vi "string parse mathematica assosiated array.vi"(7 "action":T2=enum."parse string", 10 "map IN":map{T1, dbl}(c390), 11 "String in":string="8061 -> <|\n\"\\[Zeta]\" -> 0.029251354442, \n\"\\[Tau]1\" -> 0.014634751206, \n\"\\[Tau]S\" -> 0.003873958746, \n\"\\[Tau]N\" -> 0.000007000487,\n\"\\[Tau]C\" -> 0.006827504775,\n\"\\[Kappa]0\" -> 0.000000056438,\n\"mm1\" -> 0.000000000000,\n\"mm2\" -> 0.000000000000,\n\"mm3\" -> 0.000000000000,\n\"T\" ->  5.820000000000,\n\"B\" -> 12.000000000000,\n\"\\[Theta]\" -> 0.000000000000\n|>, \n\n ") -> (2 "Map OUT":map{T1, dbl}(c390), 3 "String OUT":string="8061 -> <|\n\"\\[Zeta]\" -> 0.029251354442, \n\"\\[Tau]1\" -> 0.014634751206, \n\"\\[Tau]S\" -> 0.003873958746, \n\"\\[Tau]N\" -> 0.000007000487,\n\"\\[Tau]C\" -> 0.006827504775,\n\"\\[Kappa]0\" -> 0.000000056438,\n\"mm1\" -> 0.000000000000,\n\"mm2\" -> 0.000000000000,\n\"mm3\" -> 0.000000000000,\n\"T\" ->  5.820000000000,\n\"B\" -> 12.000000000000,\n\"\\[Theta]\" -> 0.000000000000\n|>, \n\n ")   [LabVIEW 2021]
uses:
  3-lorentzian-parameters.ctl
  mathematica string map action.ctl
  <vilib>/regexp/Match Regular Expression.xnode
panel:
  out "Map 2":map{T1, string}(c390)
  out "Map":map{T1, string}(c390)
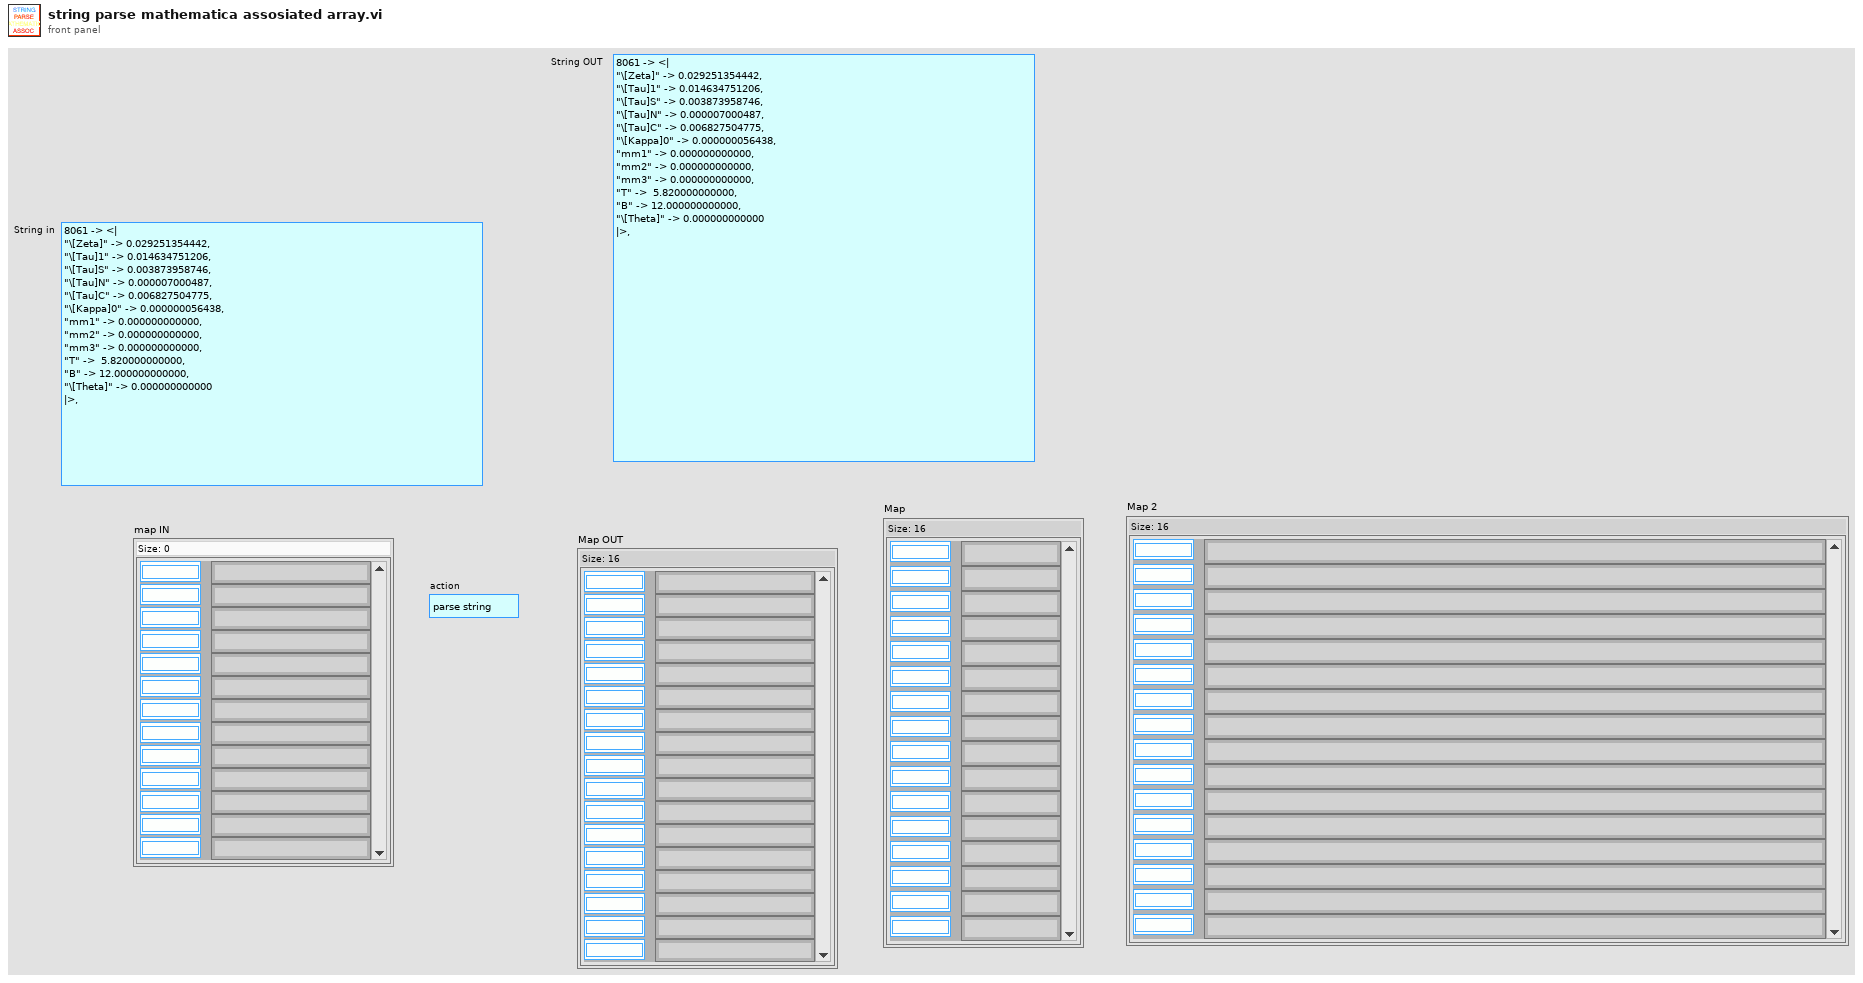
[diagram p1: front panel]
types:
  T1 = typedef "3-lorentzian-parameters.ctl" = enum16{"ζ", "τ1", "τS", "τN", "τC", "κ0", "m1", "m2", "m3", "T (K)", "B (T)", "θ (deg)", "side (S|R)", "set of (B|T)", "Re(offset)", "Im(offset)", "στ1", "στ1-", "στ1+", "στS", "στS-", "στS+"}
  T2 = typedef "mathematica string map action.ctl" = enum16{"create string", "calc m1m2m3", "parse string"}
  T3 = cluster{"keys":T1[], "regexps":string[], "labels":string[]}
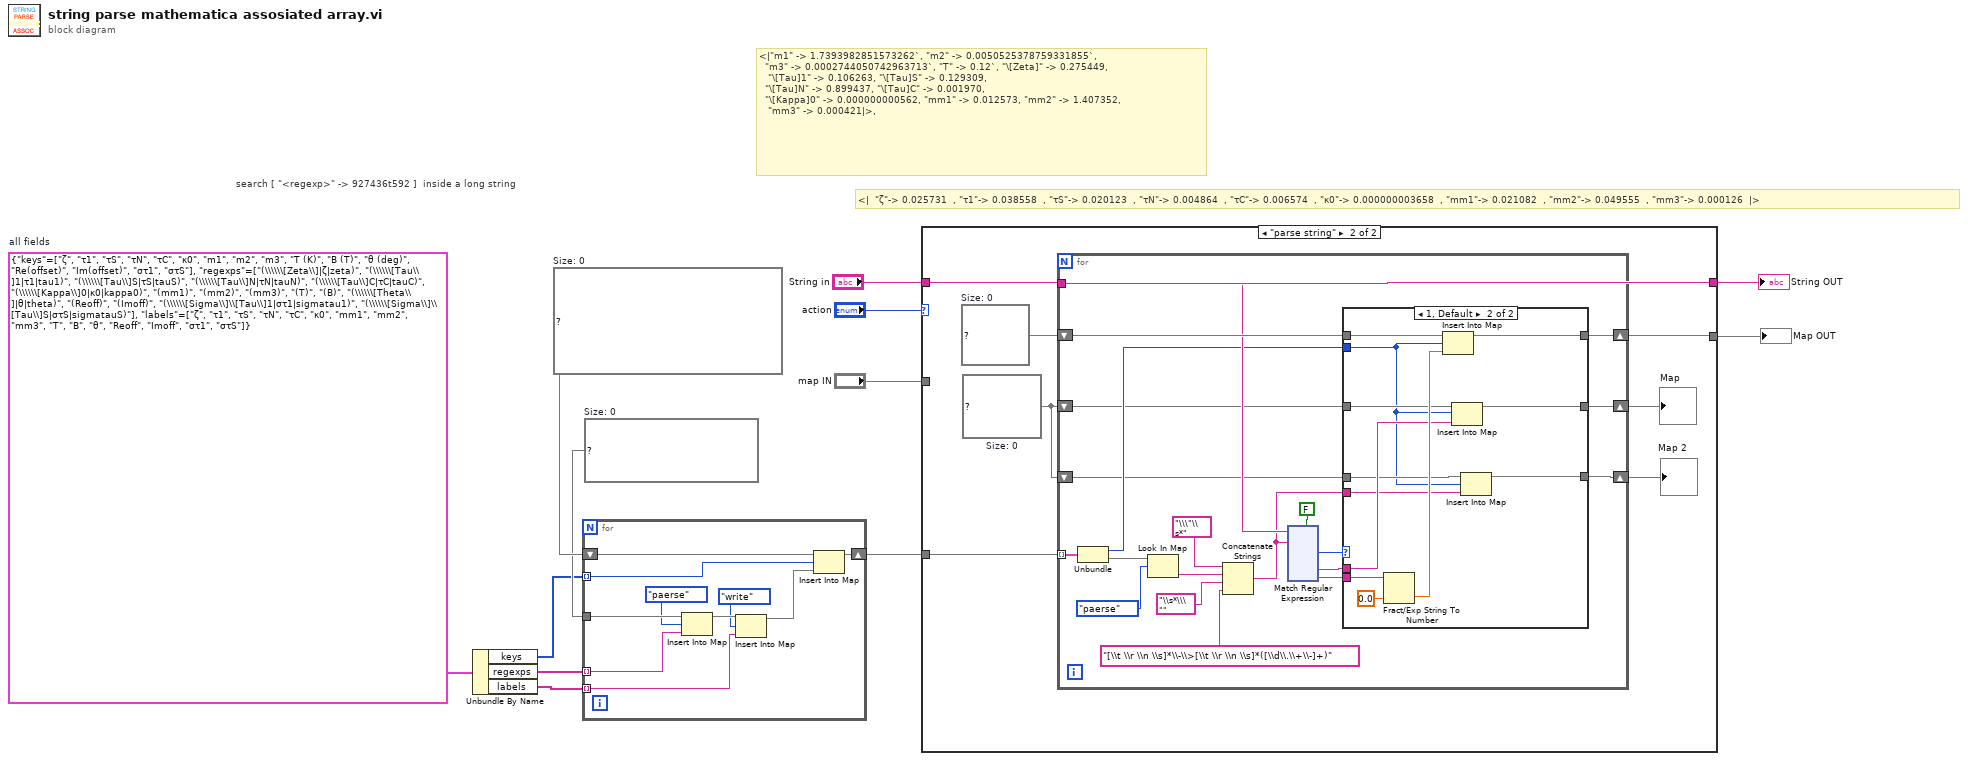
[diagram p0: block diagram]
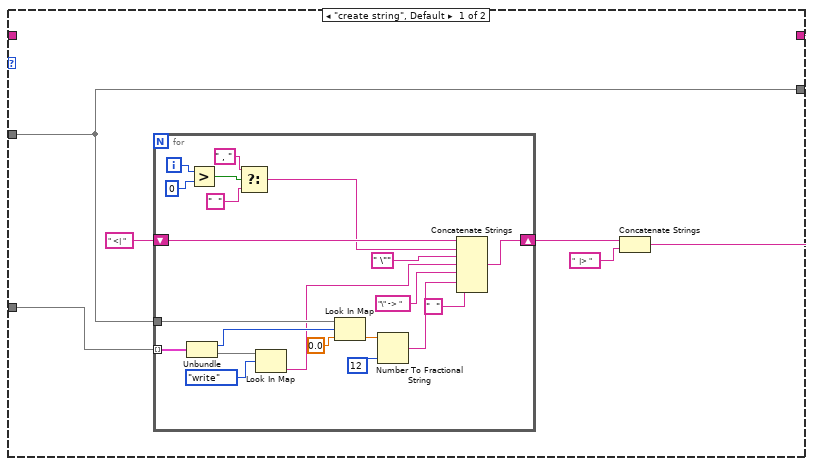
[diagram p2: hidden frame]
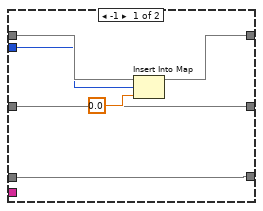
[diagram p3: hidden frame]
diagram:
  w4 = T3 {"keys"=[enum."ζ", enum."τ1", enum."τS", enum."τN", enum."τC", enum."κ0", enum."m1", enum."m2", enum."m3", enum."T (K)", enum."B (T)", enum."θ (deg)", enum."Re(offset)", enum."Im(offset)", enum."στ1", enum."στS"], "regexps"=["(\\\\\\[Zeta\\]|ζ|zeta)", "(\\\\\\[Tau\\]1|τ1|tau1)", "(\\\\\\[Tau\\]S|τS|tauS)", "(\\\\\\[Tau\\]N|τN|tauN)", "(\\\\\\[Tau\\]C|τC|tauC)", "(\\\\\\[Kappa\\]0|κ0|kappa0)", "(mm1)", "(mm2)", "(mm3)", "(T)", "(B)", "(\\\\\\[Theta\\]|θ|theta)", "(Reoff)", "(Imoff)", "(\\\\\\[Sigma\\]\\[Tau\\]1|στ1|sigmatau1)", "(\\\\\\[Sigma\\]\\[Tau\\]S|στS|sigmatauS)"], "labels"=["ζ", "τ1", "τS", "τN", "τC", "κ0", "mm1", "mm2", "mm3", "T", "B", "θ", "Reoff", "Imoff", "στ1", "στS"]}  # all fields
  w7 = map{enum16{"paerse", "write"}, string} {}  # Size: 0
  w8 = map{T1, map{enum16{"paerse", "write"}, string}} {}  # Size: 0
  # "search [ \"<regexp>\" -> 927436t592 ]  inside a long string"
  # "<|\"m1\" -> 1.7393982851573262`, \"m2\" -> 0.0050525378759331855`, \n  \"m3\" -> 0.0002744050742963713`, \"T\" -> 0.12`, \"\\[Zeta]\" -> 0.275449,\n   \"\\[Tau]1\" -> 0.106263, \"\\[Tau]S\" -> 0.129309, \n  \"\\[Tau]N\" -> 0.899437, \"\\[Tau]C\" -> 0.001970, \n  \"\\[Kappa]0\" -> 0.000000000562, \"mm1\" -> 0.012573, \"mm2\" -> 1.407352,\n   \"mm3\" -> 0.000421|>,"
  # "<|  \"ζ\"-> 0.025731  , \"τ1\"-> 0.038558  , \"τS\"-> 0.020123  , \"τN\"-> 0.004864  , \"τC\"-> 0.006574  , \"κ0\"-> 0.000000003658  , \"mm1\"-> 0.021082  , \"mm2\"-> 0.049555  , \"mm3\"-> 0.000126  |>"
  n1 = Unbundle By Name(w4) -> ("keys"=w3:T1[], "regexps"=w2:string[], "labels"=w1:string[])
  n2 = for {
    tunnel: w3 -> [w20] mode=indexing
    shift-right: [w21] -> w6
    shift-left: w8 -> [w22]
    tunnel: w7 -> [w19]
    tunnel: w2 -> [w13] mode=indexing
    tunnel: w1 -> [w14] mode=indexing
    n3 = Insert Into Map(map in=w19, key=enum16{"paerse", "write"}."paerse", value=w13) -> (map out=w18:map{enum16{"paerse", "write"}, string})  [unwired: 2 out]
    n4 = Insert Into Map(map in=w18, key=enum16{"paerse", "write"}."write", value=w14) -> (map out=w17:map{enum16{"paerse", "write"}, string})  [unwired: 2 out]
    n5 = Insert Into Map(map in=w22, key=w20, value=w17) -> (map out=w21:map{T1, map{enum16{"paerse", "write"}, string}})  [unwired: 2 out]
  }
  n6 = case shown="\"parse string\"" "action" {
    tunnel: "String in" -> [_ w54]
    tunnel: [w24 w55] -> w5
    tunnel: [w25 w54] -> w10
    tunnel: w6 -> [w23 w53]
    tunnel: "map IN" -> [w24 _]
    frame "create string", Default {
      n7 = for {
        shift-right: [w49] -> w27
        shift-left: " <| " -> [w45]
        tunnel: w23 -> [w43] mode=indexing
        tunnel: w24 -> [w48]
        i -> [w39]
        n8 = Unbundle(w43) -> ("what"=w47:T1, w42:map{enum16{"paerse", "write"}, string})
        n9 = Greater?(x=w39, y=0) -> (0:w37:bool)
        n10 = Select(t=" , ", s=w37, f="  ") -> (s? t:f=w34:string)
        n11 = Look In Map(map=w42, key=enum16{"paerse", "write"}."write") -> (value=w32:string)  [unwired: 1 in, 1 out]
        n12 = Look In Map(map=w48, key=w47, default value=0.0) -> (value=w46:dbl)  [unwired: 1 out]
        n13 = Number To Fractional String(number=w46, precision (6)=i16 12) -> (F-format string=w30:string)  [unwired: 2 in]
        n14 = Concatenate Strings(w45, w34, " \"", w32, "\" -> ", w30, "  ") -> (w49:string)
      }
      n15 = Concatenate Strings(w27, "  |> ") -> (w25:string)
    }
    frame "parse string" {
      w51 = map{T1, string} {}  # Size: 0
      w56 = map{T1, dbl} {}  # Size: 0
      n16 = for {
        tunnel: w53 -> [w75] mode=indexing
        tunnel: w54 -> [w68]
        shift-right: [w74] -> w55
        shift-left: w56 -> [w76]
        shift-right: [w65] -> w52
        shift-left: w51 -> [w66]
        shift-right: [w62] -> w50
        shift-left: w51 -> [w63]
        n17 = Unbundle(w75) -> ("what"=w67:T1, w73:map{enum16{"paerse", "write"}, string})
        n18 = Look In Map(map=w73, key=enum16{"paerse", "write"}."paerse") -> (value=w61:string)  [unwired: 1 in, 1 out]
        n19 = Concatenate Strings("\\\"\\s*" ("format string"), w61, "\\s*\\\"" ("format string"), "[\\t \\r \\n \\s]*\\-\\>[\\t \\r \\n \\s]*([\\d\\.\\+\\-]+)" ("format string")) -> (w58:string)
        n20 = xnode "Match Regular Expression"("input string"=w68, "regular expression"=w58, "multiline? (F)"=FALSE) -> ("offset past match"=w69:i32, "submatch 1"=w64:string, "submatch 2"=w70:string)  [unwired: 3 in, 4 out]
        n21 = case shown="1, Default" w69 {
          tunnel: w76 -> [w82 w94]
          tunnel: w67 -> [w80 w84]
          tunnel: [w81 w92] -> w74
          tunnel: w70 -> [_ w91]
          tunnel: w66 -> [w78 w90]
          tunnel: [w78 w89] -> w65
          tunnel: w64 -> [_ w88]
          tunnel: w63 -> [w77 w86]
          tunnel: [w77 w85] -> w62
          tunnel: w58 -> [_ w83]
          frame -1 {
            n22 = Insert Into Map(map in=w82, key=w80, value=0.0) -> (map out=w81:map{T1, dbl})  [unwired: 2 out]
          }
          frame 1, Default {
            n23 = Fract/Exp String To Number(string=w91, default (0 dbl)=0.0 ("default (0 DBL)")) -> (number=w93:dbl)  [unwired: 2 in, 1 out]
            n24 = Insert Into Map(map in=w94, key=w84, value=w93) -> (map out=w92:map{T1, dbl})  [unwired: 2 out]
            n25 = Insert Into Map(map in=w90, key=w84, value=w88) -> (map out=w89:map{T1, string})  [unwired: 2 out]
            n26 = Insert Into Map(map in=w86, key=w84, value=w83) -> (map out=w85:map{T1, string})  [unwired: 2 out]
          }
        }
      }
      "Map" <- w52
      "Map 2" <- w50
    }
  }
  "Map OUT" <- w5
  "String OUT" <- w10
